vi "Acquire Temperature.vi"(8 "error in (no error)":errorcluster, 11 "ARS-0220 in":refnum<class "ARS-0220.lvclass">) -> (0 "error out":errorcluster, 2 "Temp Data":T1, 3 "ARS-0220 out":refnum<class "ARS-0220.lvclass">)   [LabVIEW 2021, in "Environment Chamber.lvlib" / "ARS-0220.lvclass"]
uses:
  ARS-0220.lvclass
  ARS-0220.lvclass/ARS-0220.ctl
  Support Libraries/Climatic Chamber/Climatic Chamber.lvlib
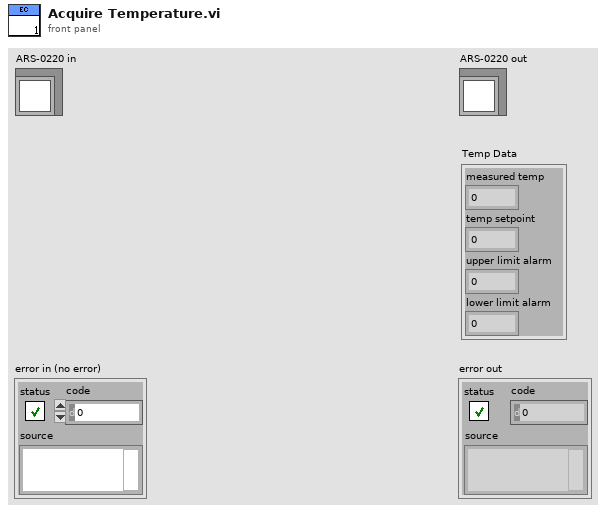
[diagram p1: front panel]
types:
  T1 = cluster{"measured temp":dbl, "temp setpoint":dbl, "upper limit alarm":dbl, "lower limit alarm":dbl}
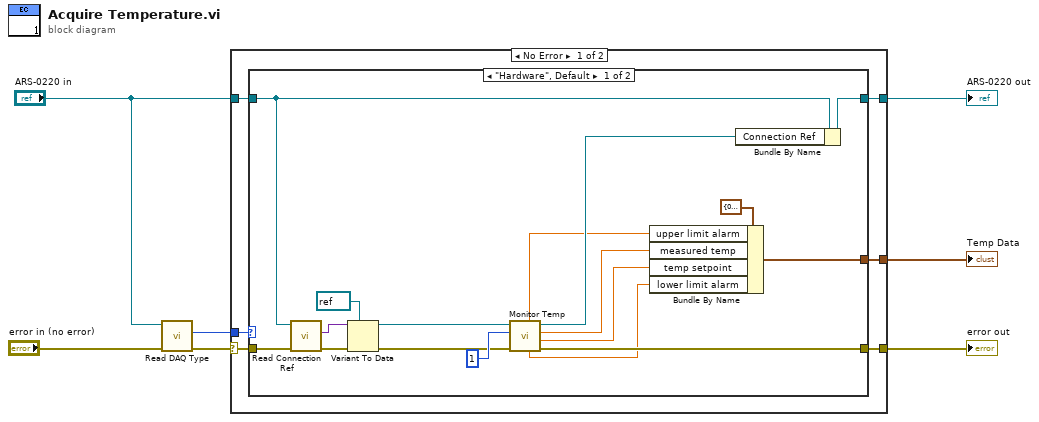
[diagram p0: block diagram]
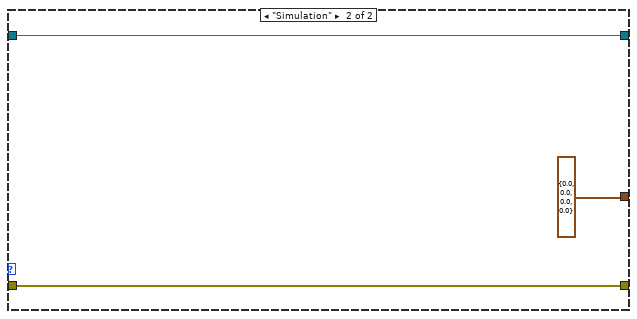
[diagram p2: hidden frame]
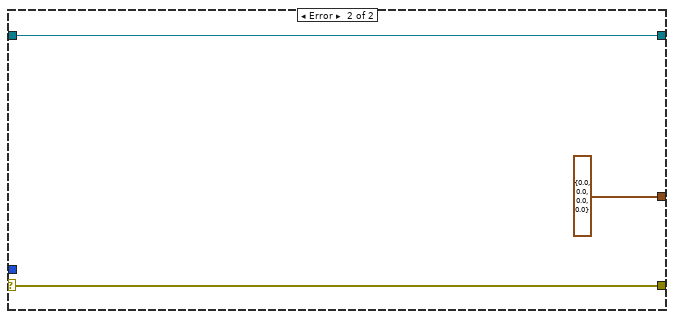
[diagram p3: hidden frame]
diagram:
  n1 = call "Read DAQ Type.vi"("error in (no error)"="error in (no error)", "ARS-0220 in"="ARS-0220 in") -> ("error out"=w6:errorcluster, "DAQ Type"=w4:enum16{"Hardware", "Simulation"})  [unwired: 7 in, 1 out]
  n2 = case shown="No Error" w6 {
    selector: w6 -> [w12 w35]
    tunnel: "ARS-0220 in" -> [w11 w36]
    tunnel: w4 -> [w13 _]
    tunnel: [w10 w36] -> w3
    tunnel: [w9 w35] -> w2
    tunnel: [w8 T1 {"measured temp"=0.0, "temp setpoint"=0.0, "upper limit alarm"=0.0, "lower limit alarm"=0.0} ("Temp Data")] -> w1
    frame No Error {
      n3 = case shown="\"Hardware\", Default" w13 {
        tunnel: w12 -> [w29 w32]
        tunnel: w11 -> [w27 w33]
        tunnel: [w22 w33] -> w10
        tunnel: [w20 w32] -> w9
        tunnel: [w14 T1 {"measured temp"=0.0, "temp setpoint"=0.0, "upper limit alarm"=0.0, "lower limit alarm"=0.0} ("Temp Data")] -> w8
        frame "Hardware", Default {
          n4 = call "Read Connection Ref.vi"("error in (no error)"=w29, "ARS-0220 in"=w27) -> ("error out"=w28:errorcluster, "Connection Ref"=w25:variant)  [unwired: 7 in, 1 out]
          n5 = Variant To Data(error in=w28, type=refnum<visa-resource-name> refnum ("VISA resource name"), Variant=w25) -> (data=w23:refnum<visa-resource-name>, error out=w26:errorcluster)
          n6 = call "Monitor Temp.vi"("error in (no error)"=w26, "Address (0)"=1, "VISA resource name"=w23) -> ("error out"=w20:errorcluster, "temp setpoint"=w16:dbl, "measured temp"=w17:dbl, "VISA resource name out"=w21:refnum<visa-resource-name>, "lower limit alarm"=w15:dbl, "upper limit alarm"=w18:dbl)  [unwired: 3 in]
          n7 = Bundle By Name(cluster=T1 {"measured temp"=0.0, "temp setpoint"=0.0, "upper limit alarm"=0.0, "lower limit alarm"=0.0} ("Temp Data"), "upper limit alarm"=w18, "measured temp"=w17, "temp setpoint"=w16, "lower limit alarm"=w15) -> (w14:T1)
          n8 = Bundle By Name(cluster=w27, "Connection Ref"=w21) -> (w22:refnum<class "ARS-0220.lvclass">)
        }
        frame "Simulation" {
        }
      }
    }
    frame Error {
    }
  }
  "error out" <- w2
  "ARS-0220 out" <- w3
  "Temp Data" <- w1
